vi "Destroy.vi"(0 "reference in":refnum<class "RefferenceB.lvclass">, 11 "Error In":errorcluster) -> (4 "reference out":refnum<class "RefferenceB.lvclass">, 15 "Error Out":errorcluster)   [LabVIEW 2018, in "RefferenceB.lvclass"]
uses:
  RefferenceB.lvclass
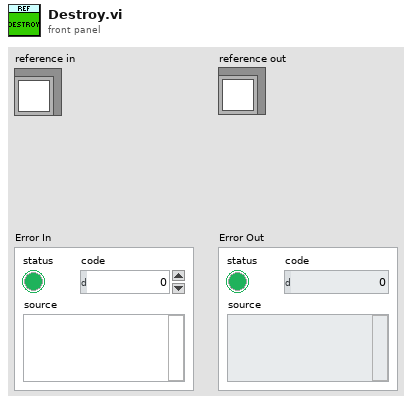
[diagram p1: front panel]
types:
  T1 = typedef "RefferenceB.lvclass/ObjectAttributes.ctl" = cluster{"Attribute1":dbl}
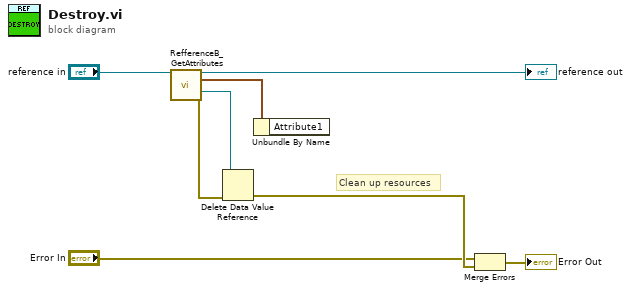
[diagram p0: block diagram]
diagram:
  # "Clean up resources"
  n1 = call "RefferenceB_GetAttributes.vi"("reference in"="reference in") -> ("reference out"=→"reference out":refnum<class "RefferenceB.lvclass">, "Data"=w3:T1, "DataRef"=w4:refnum<data-value>, "error out"=w5:errorcluster)  [unwired: 11 in]
  n2 = Delete Data Value Reference(data value reference=w4, error in=w5) -> (error out=w2:errorcluster)  [unwired: 1 out]
  n3 = Unbundle By Name(w3) -> ()  [unwired: 1 out]
  n4 = Merge Errors("Error In", w2) -> (→"Error Out":errorcluster)
